vi "set_number_of_sweeps.vi"(8 "error in (no error)":errorcluster, 10 "number of sweeps":i32, 11 "IntrinsicImagingMG091001 in":refnum<class "DataCollectionMG091001IntrinsicImaging.lvclass">) -> (0 "error out":errorcluster, 3 "IntrinsicImagingMG091001 out":refnum<class "DataCollectionMG091001IntrinsicImaging.lvclass">)   [LabVIEW 2010]
uses:
  DataCollectionMG091001IntrinsicImaging.lvclass
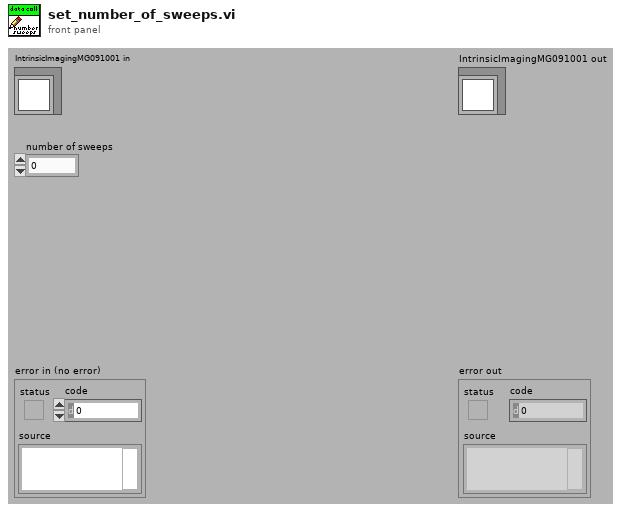
[diagram p1: front panel]
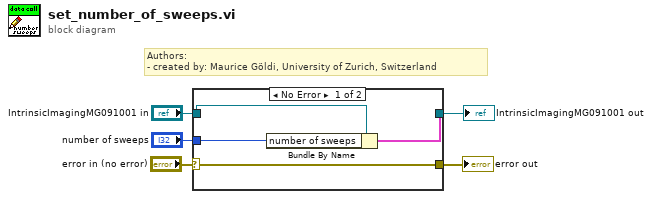
[diagram p0: block diagram]
diagram:
  # "Authors: \n- created by: Maurice Göldi, University of Zurich, Switzerland"
  n1 = case shown="No Error" "error in (no error)" {
    selector: "error in (no error)" -> [w9 w10]
    tunnel: [w9 w10] -> w4
    tunnel: [w7 w11] -> w2
    tunnel: "IntrinsicImagingMG091001 in" -> [w8 w11]
    tunnel: "number of sweeps" -> [w6 _]
    frame No Error {
      n2 = Bundle By Name(cluster=w8, "number of sweeps"=w6) -> (w7:cluster{})
    }
    frame Error {
    }
  }
  "error out" <- w4
  "IntrinsicImagingMG091001 out" <- w2
